vi "JPG_import.vi"(8 "error in (no error)":errorcluster, 10 "File name":string, 11 "File path":string) -> (0 "error out":errorcluster, 2 "new picture":picture, 3 "Complete File path":string)   [LabVIEW 2018]
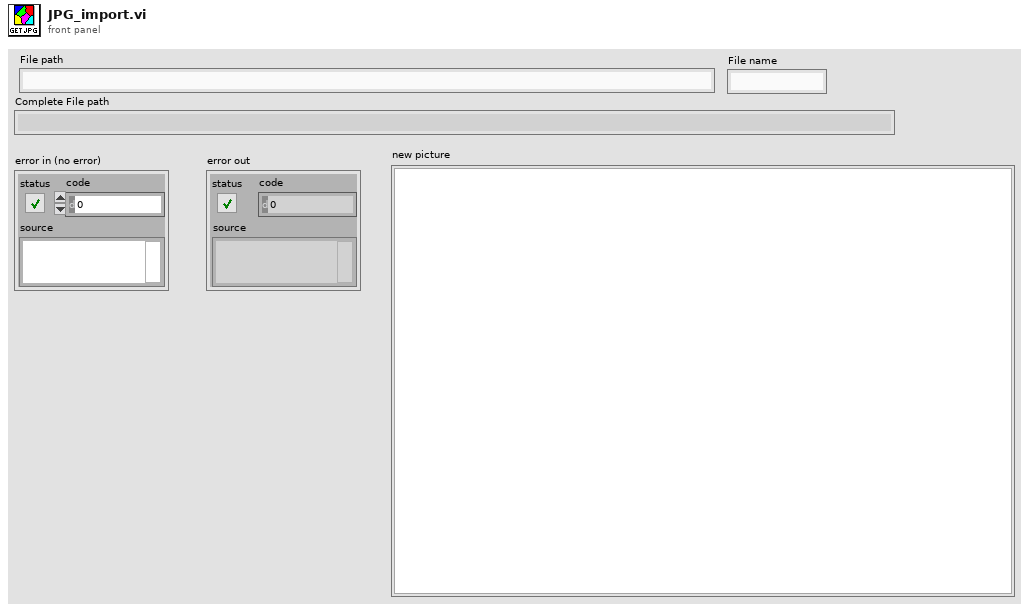
[diagram p1: front panel]
types:
  T1 = typedef "imagedata.ctl" = cluster{"image type":i32, "image depth":i32, "image":u8[], "mask":u8[], "colors":u32[], "Rectangle":cluster{"left":i16, "top":i16, "right":i16, "bottom":i16}}
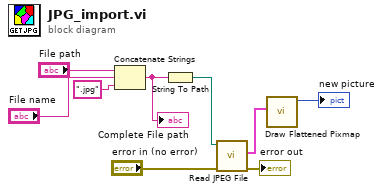
[diagram p0: block diagram]
diagram:
  n1 = Concatenate Strings("File path", "File name", ".jpg" ("string")) -> (w7:string)
  "Complete File path" <- w7
  n2 = String To Path(string=w7) -> (path=w6:path)
  n3 = call <vilib>:"Read JPEG File.vi"("error in (no error)"="error in (no error)", "path to JPEG file"=w6) -> ("error out"=→"error out":errorcluster, "image data"=w9:T1)  [unwired: 7 in, 1 out]
  n4 = call <vilib>:"Draw Flattened Pixmap.vi"("image data"=w9) -> ("new picture"=→"new picture":picture)  [unwired: 8 in]
